vi "XYZ_SHIFT.vi"() -> ()   [LabVIEW 2018]
panel:
  out "Waveform Graph":dbl[][](graph)
  out "Z SHIFT":dbl[](array[numeric])
  out "Y SHIFT":dbl[](array[numeric])
  out "X SHIFT":dbl[](array[numeric])
  in  "stop":bool
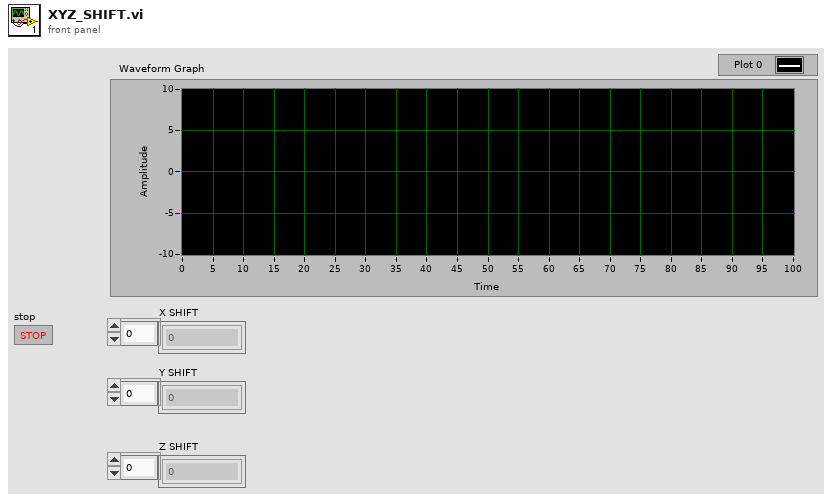
[diagram p1: front panel]
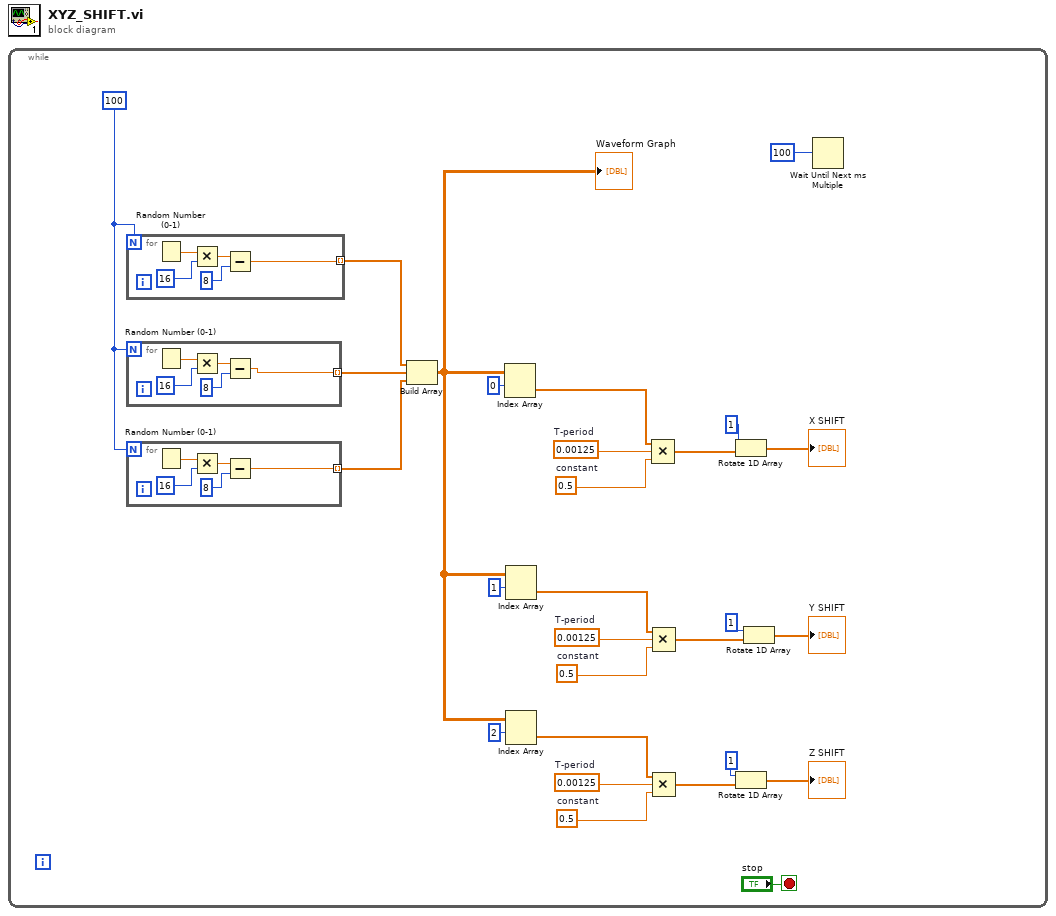
[diagram p0: block diagram]
diagram:
  n1 = while {
    stop <- "stop" stop-if-true
    w14 = 0.5  # constant
    w15 = 0.00125  # T-period
    w18 = 0.5  # constant
    w19 = 0.00125  # T-period
    w22 = 0.5  # constant
    w23 = 0.00125  # T-period
    w26 = 100
    n2 = for {
      N: w26 -> [_]
      tunnel: [w39] -> w27 mode=indexing
      n3 = Random Number (0-1)() -> (number: 0 to 1=w43:dbl)
      n4 = Multiply(x=w43, y=16) -> (x*y=w41:dbl)
      n5 = Subtract(x=w41, y=8) -> (x-y=w39:dbl)
    }
    n6 = for {
      N: w26 -> [_]
      tunnel: [w34] -> w25 mode=indexing
      n7 = Random Number (0-1)() -> (number: 0 to 1=w38:dbl)
      n8 = Multiply(x=w38, y=16) -> (x*y=w36:dbl)
      n9 = Subtract(x=w36, y=8) -> (x-y=w34:dbl)
    }
    n10 = for {
      N: w26 -> [_]
      tunnel: [w29] -> w24 mode=indexing
      n11 = Random Number (0-1)() -> (number: 0 to 1=w33:dbl)
      n12 = Multiply(x=w33, y=16) -> (x*y=w31:dbl)
      n13 = Subtract(x=w31, y=8) -> (x-y=w29:dbl)
    }
    n14 = Build Array(w27, w25, w24) -> (w3:dbl[][])
    "Waveform Graph" <- w3
    n15 = Index Array(array=w3, index (row)=0) -> (element=w20:dbl[])  [unwired: 1 in]
    n16 = Index Array(array=w3, index (row)=1) -> (element=w16:dbl[])  [unwired: 1 in]
    n17 = Index Array(array=w3, index (row)=2) -> (element=w12:dbl[])  [unwired: 1 in]
    n18 = Compound Arithmetic op=MULTIPLY(w20, w23, w22) -> (w4:dbl[])
    n19 = Compound Arithmetic op=MULTIPLY(w16, w19, w18) -> (w5:dbl[])
    n20 = Compound Arithmetic op=MULTIPLY(w12, w15, w14) -> (w8:dbl[])
    n21 = Rotate 1D Array(1:w4, 2:1) -> (0:→"X SHIFT":dbl[])
    n22 = Rotate 1D Array(1:w8, 2:1) -> (0:→"Z SHIFT":dbl[])
    n23 = Rotate 1D Array(1:w5, 2:1) -> (0:→"Y SHIFT":dbl[])
    n24 = Wait Until Next ms Multiple(millisecond multiple=100) -> ()  [unwired: 1 out]
  }
